vi "NEECA Timer.vi"(8 "error in (no error)":errorcluster, 11 "Message Queues out":T3) -> (0 "error out":errorcluster)   [LabVIEW 2023]
uses:
  Message Queue/Message Queue.lvlib
  Message Queue/Enqueue Message (Single).vi
  controls/Burner Duty Cycle.ctl
  Message Queue/Message Cluster.ctl
  Message Queue/All Message Queues.ctl
  controls/Timer Application Cluster.ctl
panel:
  out "Timer Application Data Output":T1
  in  "Debug":bool
  out "Debug":string[](array[string])
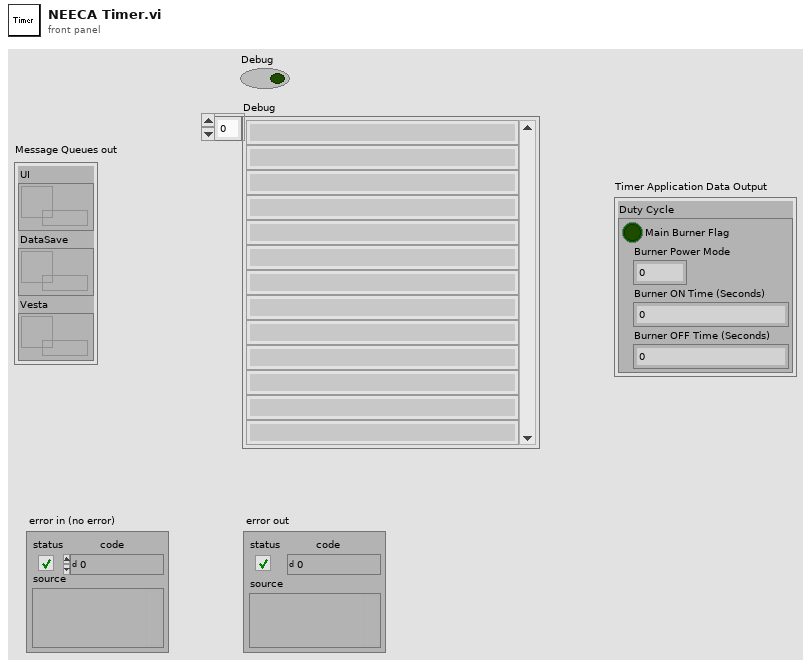
[diagram p1: front panel]
types:
  T1 = typedef "Timer Application Cluster.ctl" = cluster{"Duty Cycle":T2}
  T2 = typedef "Burner Duty Cycle.ctl" = cluster{"Burner ON Time (Seconds)":dbl, "Burner OFF Time (Seconds)":dbl, "Main Burner Flag":bool, "Burner Power Mode":u8}
  T3 = typedef "Message Queue.lvlib/All Message Queues.ctl" = cluster{"UI":refnum<queue>, "DataSave":refnum<queue>, "Vesta":refnum<queue>}
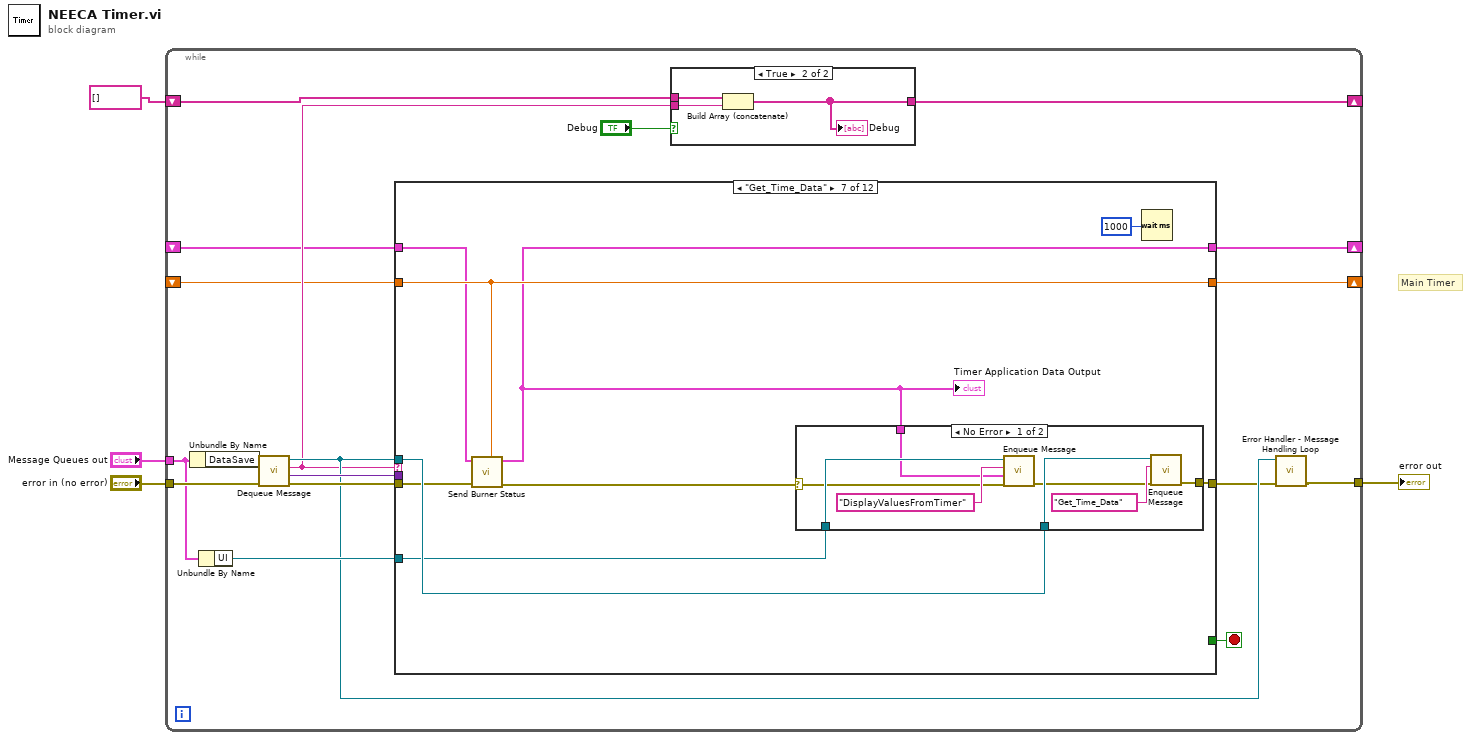
[diagram p0: block diagram]
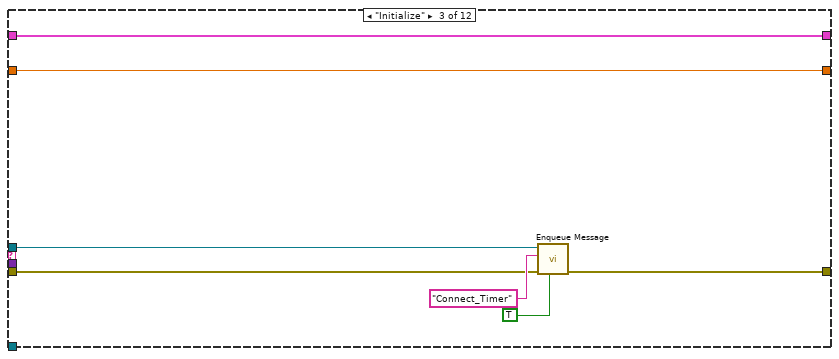
[diagram p5: hidden frame]
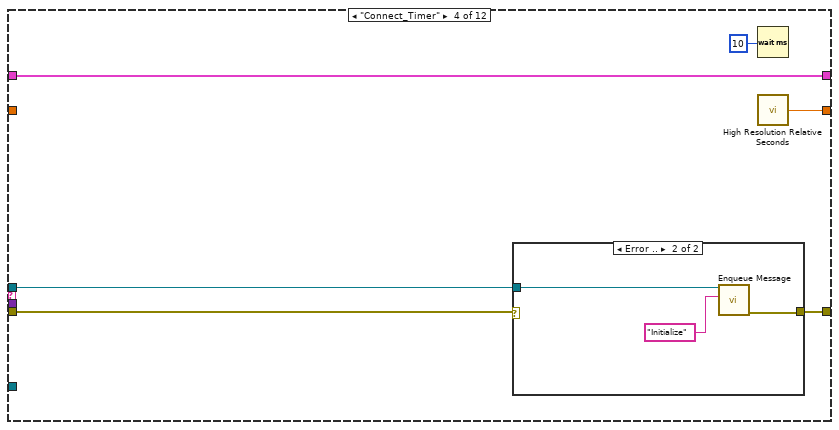
[diagram p6: hidden frame]
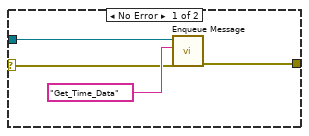
[diagram p7: hidden frame]
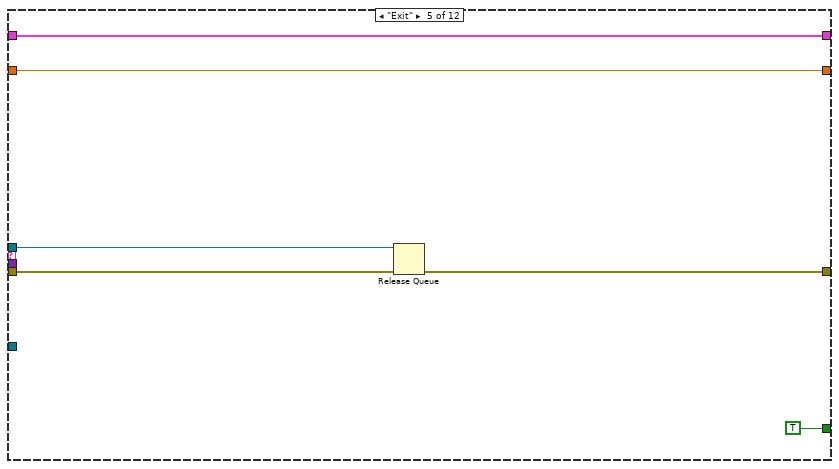
[diagram p8: hidden frame]
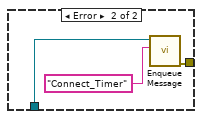
[diagram p10: hidden frame]
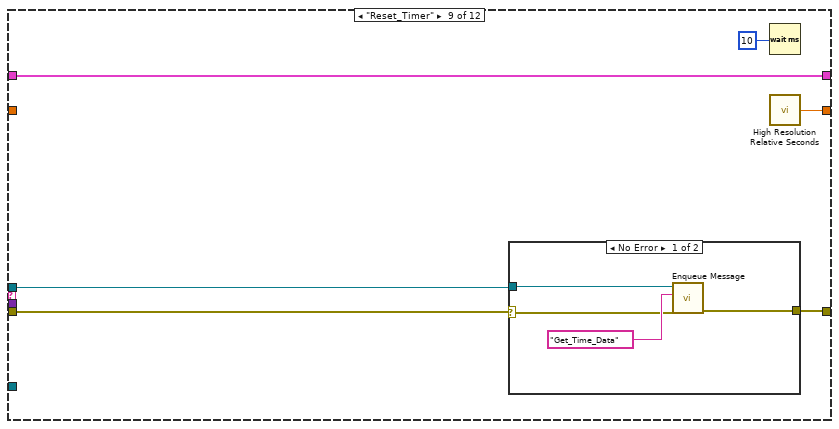
[diagram p12: hidden frame]
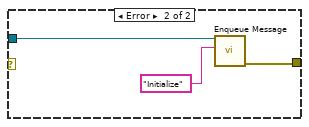
[diagram p13: hidden frame]
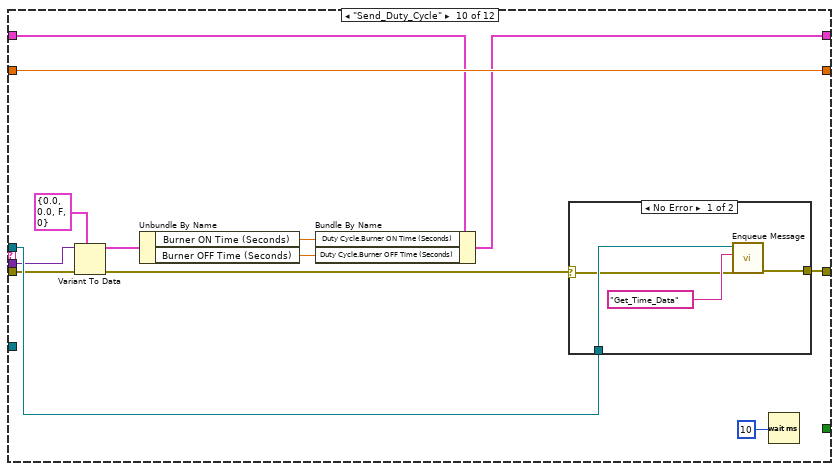
[diagram p14: hidden frame]
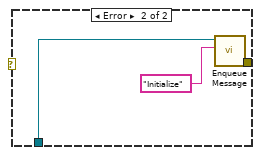
[diagram p15: hidden frame]
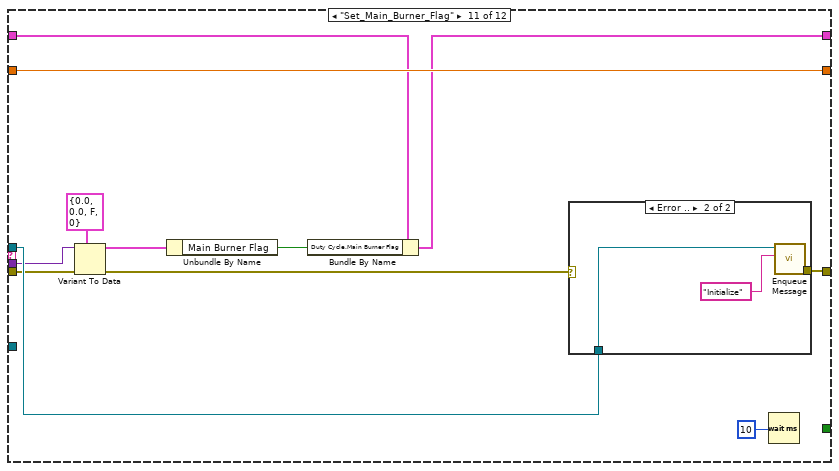
[diagram p16: hidden frame]
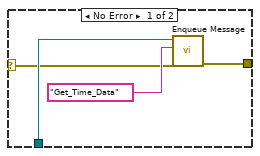
[diagram p17: hidden frame]
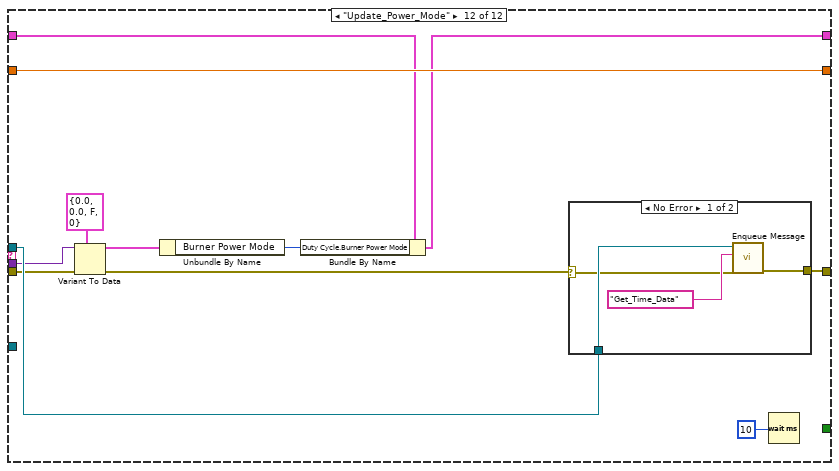
[diagram p18: hidden frame]
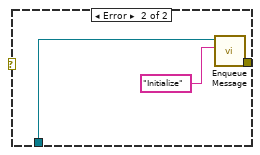
[diagram p19: hidden frame]
diagram:
  # "Main Timer"
  n1 = while {
    tunnel: "Message Queues out" -> [w15]
    tunnel: "error in (no error)" -> [w19]
    tunnel: [w11] -> w1
    shift-right: [w8] -> _
    shift-left: _ -> [w7]
    shift-right: [w16] -> _
    shift-left: string[] [] -> [w17]
    shift-right: [w5] -> _
    shift-left: _ -> [w6]
    stop <- w9 stop-if-true
    n2 = Unbundle By Name(w15) -> ("DataSave"=w22:refnum<queue>)
    n3 = Unbundle By Name(w15) -> ("UI"=w14:refnum<queue>)
    n4 = call "Dequeue Message.vi"("error in (no error)"=w19, "Message Queue"=w22) -> ("error out"=w20:errorcluster, "Message Data"=w21:variant, "Message"=w10:string, "dup Message Queue"=w13:refnum<queue>)  [unwired: 6 in]
    n5 = case shown="\"Get_Time_Data\"" w10 {
      tunnel: w13 -> [_ _ w35 w44 w57 _ w69 _ w88 w109 w128 w147]
      tunnel: w21 -> [_ _ _ _ _ _ _ _ _ w104 w123 w142]
      tunnel: w20 -> [w29 w32 w38 w43 w58 w61 w66 w84 w89 w106 w125 w144]
      tunnel: w14 -> [_ _ _ _ _ _ w64 _ _ _ _ _]
      tunnel: [w29 w32 w37 w45 w56 w61 w70 w84 w90 w110 w129 w148] -> w12
      tunnel: [_ _ _ _ TRUE _ _ _ _ _ _ _] -> w9
      tunnel: [w28 w31 w34 w42 w54 w60 w67 w83 w87 w107 w126 w145] -> w8
      tunnel: w7 -> [w28 w31 w34 _ w54 w60 w67 w83 _ w107 w126 w145]
      tunnel: w6 -> [w27 w30 w33 w40 w53 w59 w63 w82 w85 w102 w121 w140]
      tunnel: [w27 w30 w33 w40 w53 w59 w62 w82 w85 w98 w118 w138] -> w5
      frame "---------- Setup ----------" {
      }
      frame Default {
      }
      frame "Initialize" {
        n6 = call-poly "Enqueue Message.vi"("Priority Message? (F)"=TRUE, "error in (no error)"=w38, "Message"="Connect_Timer", "Message Queue"=w35) -> ("error out"=w37:errorcluster)  [unwired: 6 in, 1 out]
      }
      frame "Connect_Timer" {
        n7 = case shown="Error .." w43 {
          selector: w43 -> [w46 _]
          tunnel: [w48 w52] -> w45
          tunnel: w44 -> [w47 w50]
          frame No Error {
            n8 = call-poly "Enqueue Message.vi"("error in (no error)"=w46, "Message"="Get_Time_Data", "Message Queue"=w47) -> ("error out"=w48:errorcluster)  [unwired: 7 in, 1 out]
          }
          frame Error {
            n9 = call-poly "Enqueue Message.vi"("Message"="Initialize", "Message Queue"=w50) -> ("error out"=w52:errorcluster)  [unwired: 8 in, 1 out]
          }
        }
        n10 = Wait (ms)(milliseconds to wait=u32 10) -> ()  [unwired: 1 out]
        n11 = call <vilib>:"High Resolution Relative Seconds.vi"() -> ("relative seconds"=w42:dbl)
      }
      frame "Exit" {
        n12 = Release Queue(queue=w57, error in (no error)=w58) -> (error out=w56:errorcluster)  [unwired: 1 in, 2 out]
      }
      frame "---------- Data Collection ----------" {
      }
      frame "Get_Time_Data" {
        n13 = call "Send Burner Status.vi"("Main Timer"=w67, "error in (no error)"=w66, "Timer Application Data"=w63) -> ("error out"=w65:errorcluster, "Timer Application Data Output"=w62:T1)  [unwired: 7 in]
        "Timer Application Data Output" <- w62
        n14 = case shown="No Error" w65 {
          selector: w65 -> [w72 _]
          tunnel: [w77 w81] -> w70
          tunnel: w69 -> [w76 w79]
          tunnel: w64 -> [w74 _]
          tunnel: w62 -> [w71 _]
          frame No Error {
            n15 = call-poly "Enqueue Message.vi"("error in (no error)"=w72, "Message Data"=w71, "Message"="DisplayValuesFromTimer", "Message Queue"=w74) -> ("error out"=w75:errorcluster)  [unwired: 6 in, 1 out]
            n16 = call-poly "Enqueue Message.vi"("error in (no error)"=w75, "Message"="Get_Time_Data", "Message Queue"=w76) -> ("error out"=w77:errorcluster)  [unwired: 7 in, 1 out]
          }
          frame Error {
            n17 = call-poly "Enqueue Message.vi"("Message"="Connect_Timer", "Message Queue"=w79) -> ("error out"=w81:errorcluster)  [unwired: 8 in, 1 out]
          }
        }
        n18 = Wait (ms)(milliseconds to wait=u32 1000) -> ()  [unwired: 1 out]
      }
      frame "---------- Timer Control ----------" {
      }
      frame "Reset_Timer" {
        n19 = case shown="No Error" w89 {
          selector: w89 -> [w91 _]
          tunnel: [w93 w97] -> w90
          tunnel: w88 -> [w92 w95]
          frame No Error {
            n20 = call-poly "Enqueue Message.vi"("error in (no error)"=w91, "Message"="Get_Time_Data", "Message Queue"=w92) -> ("error out"=w93:errorcluster)  [unwired: 7 in, 1 out]
          }
          frame Error {
            n21 = call-poly "Enqueue Message.vi"("Message"="Initialize", "Message Queue"=w95) -> ("error out"=w97:errorcluster)  [unwired: 8 in, 1 out]
          }
        }
        n22 = Wait (ms)(milliseconds to wait=u32 10) -> ()  [unwired: 1 out]
        n23 = call <vilib>:"High Resolution Relative Seconds.vi"() -> ("relative seconds"=w87:dbl)
      }
      frame "Send_Duty_Cycle" {
        n24 = Variant To Data(error in=w106, type=T2 {"Burner ON Time (Seconds)"=0.0, "Burner OFF Time (Seconds)"=0.0, "Main Burner Flag"=FALSE, "Burner Power Mode"=0} ("Duty Cycle"), Variant=w104) -> (data=w101:T2, error out=w105:errorcluster)
        n25 = Unbundle By Name(w101) -> ("Burner ON Time (Seconds)"=w100:dbl, "Burner OFF Time (Seconds)"=w99:dbl)
        n26 = Bundle By Name(cluster=w102, "Duty Cycle.Burner ON Time (Seconds)"=w100, "Duty Cycle.Burner OFF Time (Seconds)"=w99) -> (w98:T1)
        n27 = case shown="No Error" w105 {
          selector: w105 -> [w111 _]
          tunnel: [w113 w117] -> w110
          tunnel: w109 -> [w112 w115]
          frame No Error {
            n28 = call-poly "Enqueue Message.vi"("error in (no error)"=w111, "Message"="Get_Time_Data", "Message Queue"=w112) -> ("error out"=w113:errorcluster)  [unwired: 7 in, 1 out]
          }
          frame Error {
            n29 = call-poly "Enqueue Message.vi"("Message"="Initialize", "Message Queue"=w115) -> ("error out"=w117:errorcluster)  [unwired: 8 in, 1 out]
          }
        }
        n30 = Wait (ms)(milliseconds to wait=u32 10) -> ()  [unwired: 1 out]
      }
      frame "Set_Main_Burner_Flag" {
        n31 = Variant To Data(error in=w125, type=T2 {"Burner ON Time (Seconds)"=0.0, "Burner OFF Time (Seconds)"=0.0, "Main Burner Flag"=FALSE, "Burner Power Mode"=0} ("Duty Cycle"), Variant=w123) -> (data=w120:T2, error out=w124:errorcluster)
        n32 = Unbundle By Name(w120) -> ("Main Burner Flag"=w119:bool)
        n33 = Bundle By Name(cluster=w121, "Duty Cycle.Main Burner Flag"=w119) -> (w118:T1)
        n34 = case shown="Error .." w124 {
          selector: w124 -> [w130 _]
          tunnel: [w132 w136] -> w129
          tunnel: w128 -> [w131 w134]
          frame No Error {
            n35 = call-poly "Enqueue Message.vi"("error in (no error)"=w130, "Message"="Get_Time_Data", "Message Queue"=w131) -> ("error out"=w132:errorcluster)  [unwired: 7 in, 1 out]
          }
          frame Error {
            n36 = call-poly "Enqueue Message.vi"("Message"="Initialize", "Message Queue"=w134) -> ("error out"=w136:errorcluster)  [unwired: 8 in, 1 out]
          }
        }
        n37 = Wait (ms)(milliseconds to wait=u32 10) -> ()  [unwired: 1 out]
      }
      frame "Update_Power_Mode" {
        n38 = Variant To Data(error in=w144, type=T2 {"Burner ON Time (Seconds)"=0.0, "Burner OFF Time (Seconds)"=0.0, "Main Burner Flag"=FALSE, "Burner Power Mode"=0} ("Duty Cycle"), Variant=w142) -> (data=w139:T2, error out=w143:errorcluster)
        n39 = Unbundle By Name(w139) -> ("Burner Power Mode"=w137:u8)
        n40 = Bundle By Name(cluster=w140, "Duty Cycle.Burner Power Mode"=w137) -> (w138:T1)
        n41 = case shown="No Error" w143 {
          selector: w143 -> [w149 _]
          tunnel: [w151 w155] -> w148
          tunnel: w147 -> [w150 w153]
          frame No Error {
            n42 = call-poly "Enqueue Message.vi"("error in (no error)"=w149, "Message"="Get_Time_Data", "Message Queue"=w150) -> ("error out"=w151:errorcluster)  [unwired: 7 in, 1 out]
          }
          frame Error {
            n43 = call-poly "Enqueue Message.vi"("Message"="Initialize", "Message Queue"=w153) -> ("error out"=w155:errorcluster)  [unwired: 8 in, 1 out]
          }
        }
        n44 = Wait (ms)(milliseconds to wait=u32 10) -> ()  [unwired: 1 out]
      }
    }
    n45 = case shown="True" "Debug" {
      tunnel: w10 -> [_ w26]
      tunnel: w17 -> [w23 w25]
      tunnel: [w23 w24] -> w16
      frame False {
      }
      frame True {
        n46 = Build Array (concatenate)(w25, w26) -> (w24:string[])
        "Debug" <- w24
      }
    }
    n47 = call "Error Handler - Message Handling Loop.vi"("error in (no error)"=w12, "Message Queue"=w13) -> ("dup error in"=w11:errorcluster)  [unwired: 8 in, 1 out]
  }
  "error out" <- w1
